vi "Browse UI.vi"(7 "Current Strings and Values":T1, 8 "error in (no error)":errorcluster, 10 "Current Value":string, 11 "Dynamic Values in":refnum<class "Dynamic Values.lvclass">) -> (0 "error out":errorcluster, 1 "Cancelled?":bool, 2 "Selected Value":string, 3 "Dynamic Values out":refnum<class "Dynamic Values.lvclass">, 5 "Strings and Values []":T1)   [LabVIEW 2020, in "Dynamic Combobox.lvlib" / "Dynamic Values.lvclass"]
uses:
  Dynamic Values.lvclass
  <vilib>/Utility/miscctls.llb/LVComboBoxStrsAndValuesArrayTypeDef.ctl
panel:
  in  "Refresh":bool
  in  "Cancel":bool
  in  "OK":bool
  in  "List":i32(listbox)
  in  "Search":string
  # "Select the value below, the text input can be used to search:"
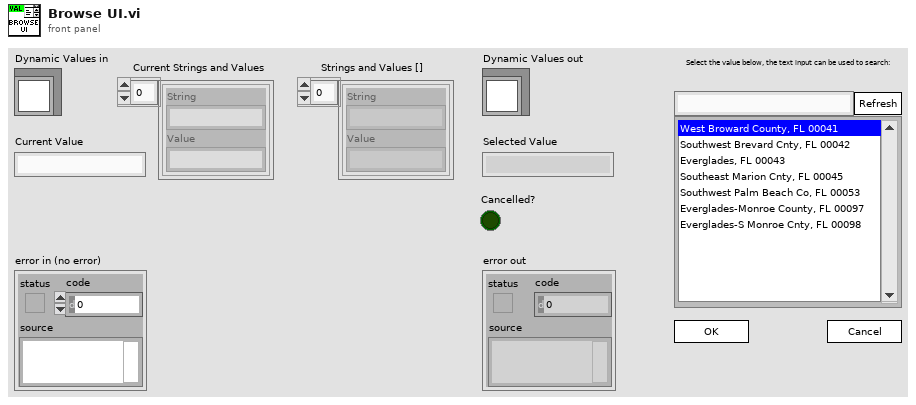
[diagram p1: front panel]
types:
  T1 = typedef "LVComboBoxStrsAndValuesArrayTypeDef.ctl" = cluster{"String":string, "Value":string}[]
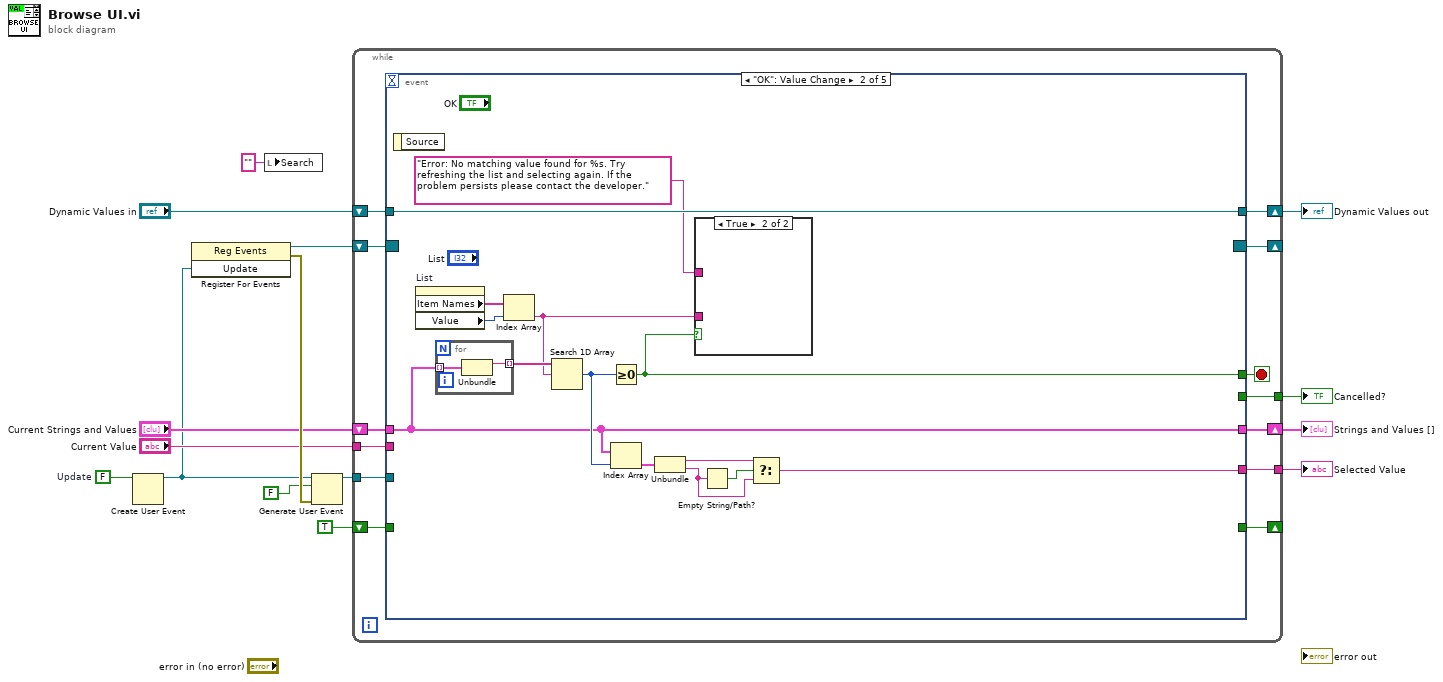
[diagram p0: block diagram]
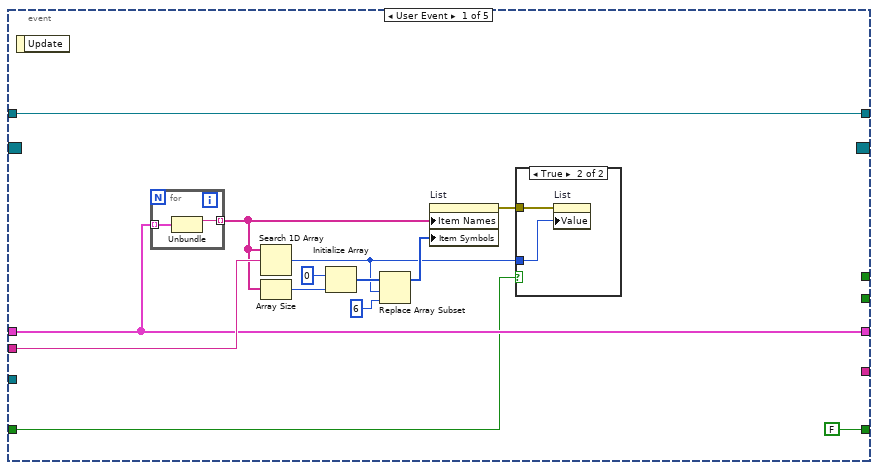
[diagram p2: hidden frame]
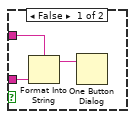
[diagram p4: hidden frame]
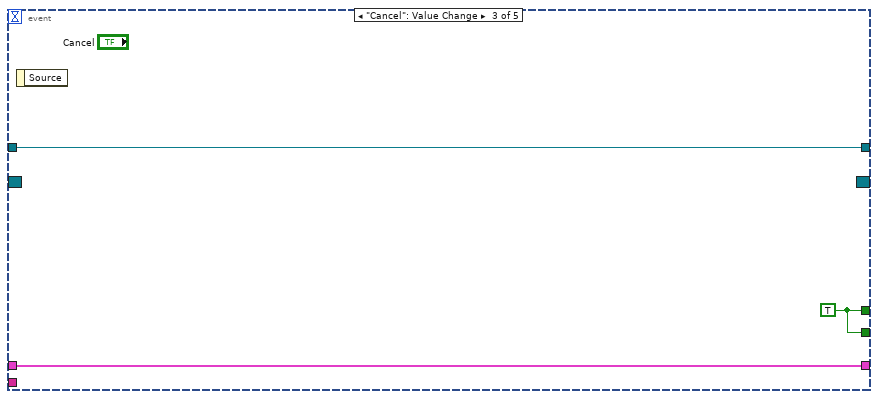
[diagram p5: hidden frame]
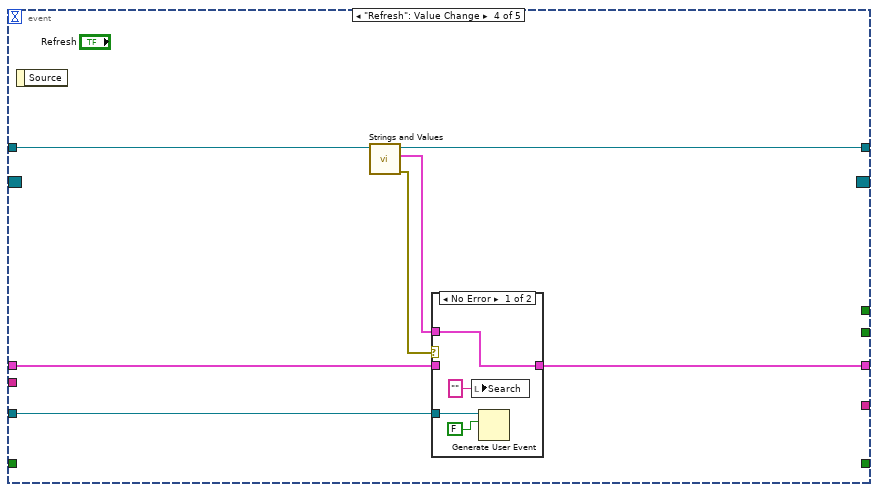
[diagram p6: hidden frame]
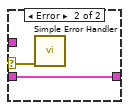
[diagram p7: hidden frame]
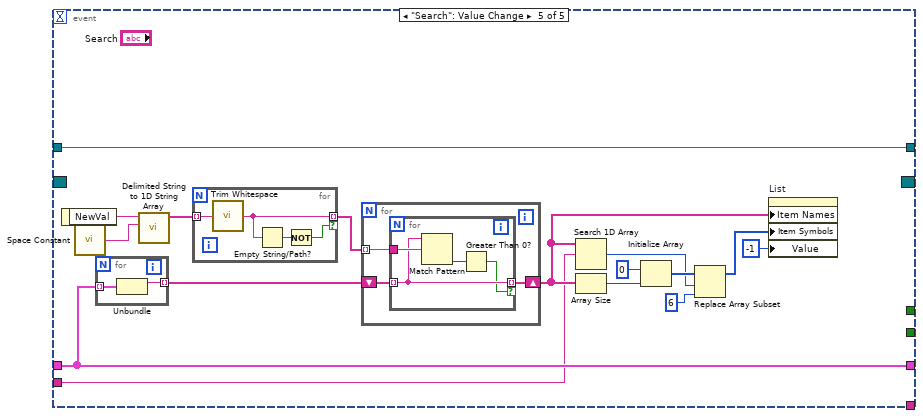
[diagram p8: hidden frame]
diagram:
  w12 = FALSE  # Update
  n1 = Create User Event(user event datatype=w12) -> (user event=w9:refnum<user-event>)  [unwired: 1 in, 1 out]
  n2 = register-events(w9) -> (reference out=w11:refnum<event-registration>, error out=w15:errorcluster)  [unwired: 2 in]
  n3 = local write "Search"("" ("Search")) -> ()
  n4 = Generate User Event(user event=w9, event data cluster=FALSE ("event data"), error in=w15) -> (user event out=w8:refnum<user-event>)  [unwired: 1 in, 1 out]
  n5 = while {
    tunnel: "Current Value" -> [w27]
    shift-right: [w24] -> w10
    shift-left: "Current Strings and Values" -> [w28]
    shift-right: [w25] -> _
    shift-left: w11 -> [w26]
    tunnel: w8 -> [w23]
    tunnel: [w21] -> w6
    shift-right: [w19] -> w4
    shift-left: "Dynamic Values in" -> [w20]
    shift-right: [w17] -> _
    shift-left: TRUE -> [w18]
    tunnel: [w16] -> w2
    stop <- w22 stop-if-true
    n6 = event shown="[1] \"OK\": Value Change" {
      selector: w26 -> [_ _ _ _ _]
      dyn-events: [_ _ _ _ _] -> w25
      timeout: _ -> [_ _ _ _ _]
      tunnel: w28 -> [w34 w53 w67 w70 w93]
      tunnel: w27 -> [w41 _ _ _ w83]
      tunnel: [w34 w53 w67 w68 w93] -> w24
      tunnel: w23 -> [_ _ _ w72 _]
      tunnel: [_ w52 w66 _ _] -> w22
      tunnel: [_ _ w66 _ _] -> w21
      tunnel: w20 -> [w33 w59 w65 w74 w96]
      tunnel: [w33 w59 w65 w73 w96] -> w19
      tunnel: w18 -> [w30 _ _ _ _]
      tunnel: [FALSE _ _ _ _] -> w17
      tunnel: [_ w46 _ _ _] -> w16
      event User Event {
        n7 = event-data() -> ()  [unwired: 1 in, 1 out]
        n8 = for {
          tunnel: w34 -> [w45] mode=indexing
          tunnel: [w44] -> w40 mode=indexing
          n9 = Unbundle(w45) -> ("String"=w44:string)  [unwired: 1 out]
        }
        n10 = Search 1D Array(1D array=w40, element=w41) -> (index of element=w32:i32)  [unwired: 1 in]
        n11 = Array Size(array=w40) -> (size(s)=w39:i32)
        n12 = Initialize Array(0 ("element"), w39) -> (w37:i32[])
        n13 = Replace Array Subset(array=w37, new element=6 ("new element/subarray"), index=w32) -> (w35:i32[])
        n14 = property on="List" class="LstBox (strict)"("Item Names"=w40, "Item Symbols"=w35) -> (error out=w31:errorcluster)  [unwired: 2 in, 1 out]
        n15 = case shown="True" w30 {
          tunnel: w32 -> [_ w43]
          tunnel: w31 -> [_ w42]
          frame False {
          }
          frame True {
            n16 = property on="List" class="LstBox (strict)"(error in=w42, "Value"=w43) -> ()  [unwired: 1 in, 2 out]
          }
        }
      }
      event "OK": Value Change {
        n17 = event-data() -> ()  [unwired: 1 in, 1 out]
        n18 = property on="List" class="LstBox (strict)"() -> ("Item Names"=w58:string[], "Value"=w57:i32)  [unwired: 2 in, 2 out]
        n19 = for {
          tunnel: w53 -> [w64] mode=indexing
          tunnel: [w63] -> w56 mode=indexing
          n20 = Unbundle(w64) -> ("String"=w63:string)  [unwired: 1 out]
        }
        n21 = Index Array(array=w58, index=w57) -> (element=w51:string)
        n22 = Search 1D Array(1D array=w56, element=w51) -> (index of element=w55:i32)  [unwired: 1 in]
        n23 = Greater Or Equal To 0?(x=w55) -> (x >= 0?=w52:bool)
        n24 = Index Array(array=w53, index=w55) -> (element=w54:cluster{"String":string, "Value":string})
        n25 = Unbundle(w54) -> ("String"=w49:string, "Value"=w47:string)
        n26 = case shown="True" w52 {
          tunnel: w51 -> [w62 _]
          tunnel: "Error: No matching value found for %s. Try refreshing the list and selecting again. If the problem persists please contact the developer." ("format string") -> [w61 _]
          frame False {
            n27 = Format Into String(format string=w61, w62) -> (resulting string=w60:string)  [unwired: 2 in, 1 out]
            n28 = One Button Dialog(message=w60) -> ()  [unwired: 1 in, 1 out]
          }
          frame True {
          }
        }
        n29 = Empty String/Path?(string/path=w47) -> (empty?=w48:bool)
        n30 = Select(t=w49, s=w48, f=w47) -> (s? t:f=w46:string)
      }
      event "Cancel": Value Change {
        w66 = TRUE
        n31 = event-data() -> ()  [unwired: 1 in, 1 out]
      }
      event "Refresh": Value Change {
        n32 = event-data() -> ()  [unwired: 1 in, 1 out]
        n33 = call-dynamic "Strings and Values.vi"("Dynamic Values in"=w74) -> ("error out"=w71:errorcluster, "Strings And Values []"=w69:T1, "Dynamic Values out"=w73:refnum<class "Dynamic Values.lvclass">)  [unwired: 8 in]
        n34 = case shown="No Error" w71 {
          selector: w71 -> [_ w79]
          tunnel: w72 -> [w77 _]
          tunnel: w70 -> [_ w80]
          tunnel: w69 -> [w76 _]
          tunnel: [w76 w80] -> w68
          frame No Error {
            n35 = local write "Search"("" ("Search")) -> ()
            n36 = Generate User Event(user event=w77, event data cluster=FALSE ("event data")) -> ()  [unwired: 2 in, 2 out]
          }
          frame Error {
            n37 = call <vilib>:"Simple Error Handler.vi"("error in (no error)"=w79) -> ()  [unwired: 4 in, 5 out]
          }
        }
      }
      event "Search": Value Change {
        n38 = event-data() -> ("NewVal"=w95:string)  [unwired: 1 in]
        n39 = call <vilib>:"Space Constant.vi"() -> ("String"=w94:string)
        n40 = for {
          tunnel: w93 -> [w109] mode=indexing
          tunnel: [w108] -> w92 mode=indexing
          n41 = Unbundle(w109) -> ("String"=w108:string)  [unwired: 1 out]
        }
        n42 = call <vilib>:"Delimited String to 1D String Array.vi"("delimiter"=w94, "delimited string"=w95) -> ("string array"=w82:string[])  [unwired: 9 in]
        n43 = for {
          tunnel: w82 -> [w100] mode=indexing
          tunnel: [w99] -> w81 mode=indexing if=w97
          n44 = call <vilib>:"Trim Whitespace.vi"("string"=w100) -> ("trimmed string"=w99:string)  [unwired: 1 in]
          n45 = Empty String/Path?(string/path=w99) -> (empty?=w98:bool)
          n46 = Not(x=w98) -> (.not. x?=w97:bool)
        }
        n47 = for {
          shift-right: [w101] -> w84
          shift-left: w92 -> [w103]
          tunnel: w81 -> [w102] mode=indexing
          n48 = for {
            tunnel: w103 -> [w106] mode=indexing
            tunnel: [w106] -> w101 mode=indexing if=w104
            tunnel: w102 -> [w107]
            n49 = Match Pattern(string=w106, regular expression=w107) -> (offset past match=w105:i32)  [unwired: 1 in, 3 out]
            n50 = Greater Than 0?(x=w105) -> (x > 0?=w104:bool)
          }
        }
        n51 = Search 1D Array(1D array=w84, element=w83) -> (index of element=w88:i32)  [unwired: 1 in]
        n52 = Array Size(array=w84) -> (size(s)=w91:i32)
        n53 = Initialize Array(0 ("element"), w91) -> (w90:i32[])
        n54 = Replace Array Subset(array=w90, new element=6 ("new element/subarray"), index=w88) -> (w89:i32[])
        n55 = property on="List" class="LstBox (strict)"("Item Names"=w84, "Item Symbols"=w89, "Value"=-1 ("List")) -> ()  [unwired: 2 in, 2 out]
      }
    }
  }
  "Dynamic Values out" <- w4
  "Selected Value" <- w2
  "Cancelled?" <- w6
  "Strings and Values []" <- w10
